vi "2nd_Order_System.vi"() -> ()   [LabVIEW 2012]
uses:
  2nd_Order_TD.ctl
  <vilib>/Analysis/1siggen.llb/Ramp Pattern by Samples.vi
  <vilib>/gmath/zero.llb/nD Nonlinear System Single Solution (VI).vi
  <vilib>/Analysis/NI_AALBase.lvlib
  <vilib>/Analysis/NI_AALPro.lvlib
  <vilib>/gmath/NI_Gmath.lvlib
panel:
  out "Phase 2":T1(graph)
  out "Magnitude 2":cluster{"Ramp Pattern":dbl[], dbl[]}[](graph)
  in  "zeta max":dbl
  in  "zeta min":dbl
  out "Phase":cluster{dbl[], dbl[]}[](graph)
  out "Magnitude":cluster{"Ramp Pattern":dbl[], dbl[]}[](graph)
  in  "omega_h":dbl
  # "This Vi computes a 2nd order system response using two methods.  Method 1 uses the linear transfer function to compute the bode plot.  Method 2 uses an iterative proceedure to find the roos of the transfer function when the RHS is set to zero.  This is so that a the frequency response of a non-linear transfer function can be calculated."
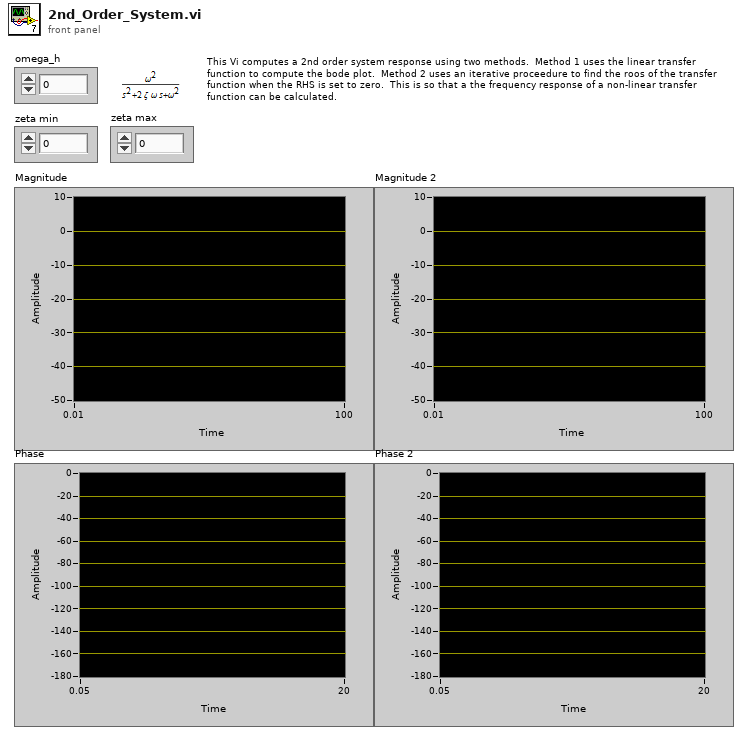
[diagram p1: front panel]
types:
  T1 = cluster{"Ramp Pattern":dbl[], "Unwrapped Phase":dbl[]}[]
  T2 = cluster{"Ramp Pattern":dbl[], "Unwrapped Phase":dbl[]}
  T3 = typedef "2nd_Order_TD.ctl" = cluster{"omega_h":dbl, "zeta":dbl, "omega":dbl}
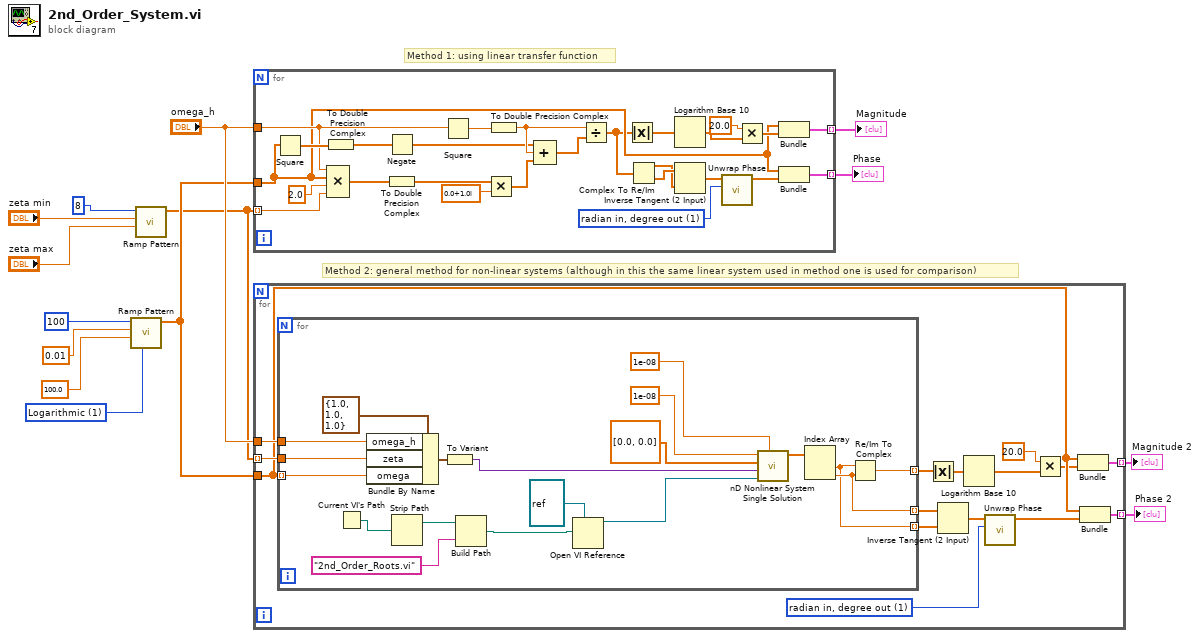
[diagram p0: block diagram]
diagram:
  w9 = u16 1 items=["Linear", "Logarithmic"] ("type")
  # "Method 2: general method for non-linear systems (although in this the same linear system used in method one is used for comparison)"
  # "Method 1: using linear transfer function"
  n1 = call-poly <vilib>:"Ramp Pattern.vi"("type"=w9, "start"=100.0, "end"=0.01, "samples"=100) -> ("Ramp Pattern"=w2:dbl[])  [unwired: 6 in, 1 out]
  n2 = call-poly <vilib>:"Ramp Pattern.vi"("start"="zeta max", "end"="zeta min", "samples"=8) -> ("Ramp Pattern"=w1:dbl[])  [unwired: 7 in, 1 out]
  n3 = for {
    tunnel: [w40] -> w14 mode=indexing
    tunnel: w1 -> [w31] mode=indexing
    tunnel: [w22] -> w12 mode=indexing
    tunnel: "omega_h" -> [w18]
    tunnel: w2 -> [w17]
    w19 = 1 items=["radian in, radian out", "radian in, degree out", "degree in, degree out", "degree in, radian out"] ("phase unit")
    n4 = Square(x=w17) -> (x^2=w30:dbl[])
    n5 = To Double Precision Complex(1:w30) -> (0:w34:cdb[])
    n6 = Compound Arithmetic op=MULTIPLY(w18, w17, 2.0 ("value"), w31) -> (w28:dbl[])
    n7 = Negate(x=w34) -> (-x=w29:cdb[])
    n8 = To Double Precision Complex(1:w28) -> (0:w27:cdb[])
    n9 = Square(x=w18) -> (x^2=w36:dbl)
    n10 = Multiply(x=w27, y=cdb 0.0+1.0i) -> (x*y=w25:cdb[])
    n11 = To Double Precision Complex(1:w36) -> (0:w35:cdb)
    n12 = Compound Arithmetic op=ADD(w29, w35, w25) -> (w39:cdb[])
    n13 = Divide(x=w35, y=w39) -> (x/y=w15:cdb[])
    n14 = Absolute Value(x=w15) -> (abs(x)=w16:dbl[])
    n15 = Complex To Re/Im(x + iy=w15) -> (x=w23:dbl[], y=w24:dbl[])
    n16 = Logarithm Base 10(1:w16) -> (0:w38:dbl[])
    n17 = Inverse Tangent (2 Input)(1:w23, 2:w24) -> (0:w21:dbl[])
    n18 = call <vilib>:"Unwrap Phase.vi"("phase unit"=w19, "Phase"=w21) -> ("Unwrapped Phase"=w20:dbl[])  [unwired: 8 in, 1 out]
    n19 = Multiply(x=20.0 ("value"), y=w38) -> (x*y=w33:dbl[])
    n20 = Bundle("Ramp Pattern"=w17, w33) -> (w40:cluster{"Ramp Pattern":dbl[], dbl[]})  [unwired: 1 in]
    n21 = Bundle("Ramp Pattern"=w17, "Unwrapped Phase"=w20) -> (w22:T2)  [unwired: 1 in]
  }
  "Magnitude" <- w14
  "Phase" <- w12
  n22 = for {
    tunnel: "omega_h" -> [w55]
    tunnel: [w54] -> w4 mode=indexing
    tunnel: [w53] -> w3 mode=indexing
    tunnel: w2 -> [w42]
    tunnel: w1 -> [w50] mode=indexing
    w52 = 1 items=["radian in, radian out", "radian in, degree out", "degree in, degree out", "degree in, radian out"] ("phase unit")
    n23 = for {
      tunnel: w55 -> [w74]
      tunnel: [w58] -> w46 mode=indexing
      tunnel: w42 -> [w65] mode=indexing
      tunnel: w50 -> [w63]
      tunnel: [w57] -> w45 mode=indexing
      tunnel: [w56] -> w44 mode=indexing
      n24 = Current VI's Path() -> (path=w62:path)
      n25 = Bundle By Name(cluster=T3 {"omega_h"=1.0, "zeta"=1.0, "omega"=1.0} ("2nd Oder TD"), "omega_h"=w74, "zeta"=w63, "omega"=w65) -> (w71:T3)
      n26 = Strip Path(path=w62) -> (stripped path=w61:path)  [unwired: 1 out]
      n27 = To Variant(anything=w71) -> (Variant=w70:variant)
      n28 = Build Path(base path=w61, name or relative path="2nd_Order_Roots.vi") -> (appended path=w59:path)
      n29 = Open VI Reference(type specifier VI Refnum (for type only)=refnum<vi> refnum, vi path=w59) -> (vi reference=w68:refnum<vi>)  [unwired: 4 in, 1 out]
      n30 = call-poly <vilib>:"nD Nonlinear System Single Solution.vi"("accuracy"=1e-08 ("h"), "F(X)"=w68, "data"=w70, "Start"=dbl[] [0.0, 0.0], "h"=1e-08) -> ("Zeroes"=w69:dbl[])  [unwired: 3 in, 3 out]
      n31 = Index Array(array=w69) -> (element #1=w56:dbl, element #2=w57:dbl)  [unwired: 2 in]
      n32 = Re/Im To Complex(1:w57, 2:w56) -> (0:w58:cdb)
    }
    n33 = Absolute Value(x=w46) -> (abs(x)=w49:dbl[])
    n34 = Inverse Tangent (2 Input)(1:w44, 2:w45) -> (0:w43:dbl[])
    n35 = Logarithm Base 10(1:w49) -> (0:w47:dbl[])
    n36 = call <vilib>:"Unwrap Phase.vi"("phase unit"=w52, "Phase"=w43) -> ("Unwrapped Phase"=w51:dbl[])  [unwired: 8 in, 1 out]
    n37 = Multiply(x=20.0 ("value"), y=w47) -> (x*y=w41:dbl[])
    n38 = Bundle("Ramp Pattern"=w42, w41) -> (w54:cluster{"Ramp Pattern":dbl[], dbl[]})  [unwired: 1 in]
    n39 = Bundle("Ramp Pattern"=w42, "Unwrapped Phase"=w51) -> (w53:T2)  [unwired: 1 in]
  }
  "Magnitude 2" <- w4
  "Phase 2" <- w3
